vi "arraystring.vi"(1 "Array In":string[](array[string]), 2 "String To Append":string) -> (0 "Array Out":string[](array[string]))   [LabVIEW 2010]
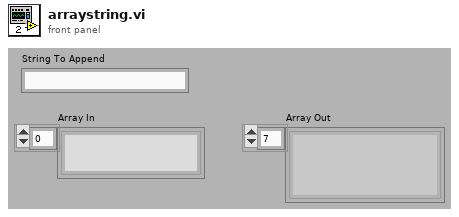
[diagram p1: front panel]
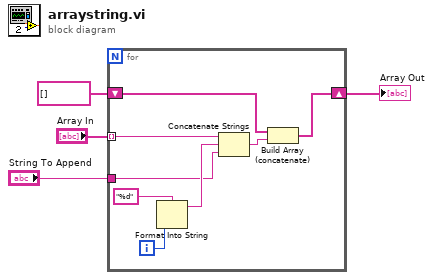
[diagram p0: block diagram]
diagram:
  n1 = for {
    tunnel: "Array In" -> [w12] mode=indexing
    shift-right: [w9] -> w2
    shift-left: string[] [] -> [w10]
    tunnel: "String To Append" -> [w6]
    i -> [w8]
    n2 = Format Into String(format string="%d", w8) -> (resulting string=w7:string)  [unwired: 2 in, 1 out]
    n3 = Concatenate Strings(w12, w7, w6) -> (w11:string)
    n4 = Build Array (concatenate)(w10, w11) -> (w9:string[])
  }
  "Array Out" <- w2
